vi "Main.vi"(7 "Is Simulated?":bool, 8 "error in":errorcluster, 9 ">>ErrorQ":refnum<queue>, 10 ">>ControllerQ":refnum<queue>, 11 ">>EventHandlers":refnum<user-event>) -> (0 "error out":errorcluster)   [LabVIEW 2020, in "ErrorHandler.lvlib"]
doc: "This is a template for creating new VIs for the owning library"
uses:
  ErrorHandler.lvlib
  Controls/Error QMsg.ctl
  Support/Controls/Project Modules.ctl
  Controller/Controls/Controller QMsg.ctl
  Support/Controls/Project Event Msg.ctl
  Support/Controls/Project Events.ctl
  Controls/Operational Loop Data.ctl
  Support/Support.lvlib
  Controls/Module Event Msg.ctl
  Controller/Controller.lvlib
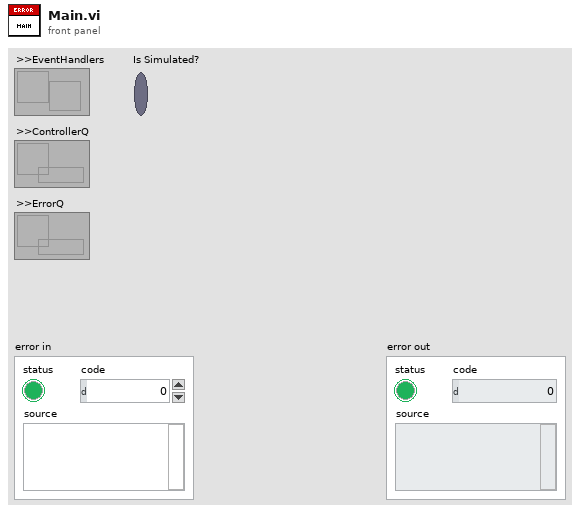
[diagram p1: front panel]
types:
  T1 = typedef "ErrorHandler.lvlib/Operational Loop Data.ctl" = cluster{"Is Simulated?":bool}
  T2 = typedef "ErrorHandler.lvlib/Module Messaging Structures.ctl" = cluster{">>EventHandlers":refnum<user-event>, ">>ErrorQ":refnum<queue>, ">>ControllerQ":refnum<queue>}
  T3 = typedef "ErrorHandler.lvlib/Module Event Msg.ctl" = cluster{"Command":string, "Data":variant}
  T4 = typedef "Support.lvlib/Project Events.ctl" = enum16{"Stop", "Initialize", "Elevator Call"}
  T5 = typedef "Controller.lvlib/Controller QMsg.ctl" = cluster{"Command":string, "Data":variant}
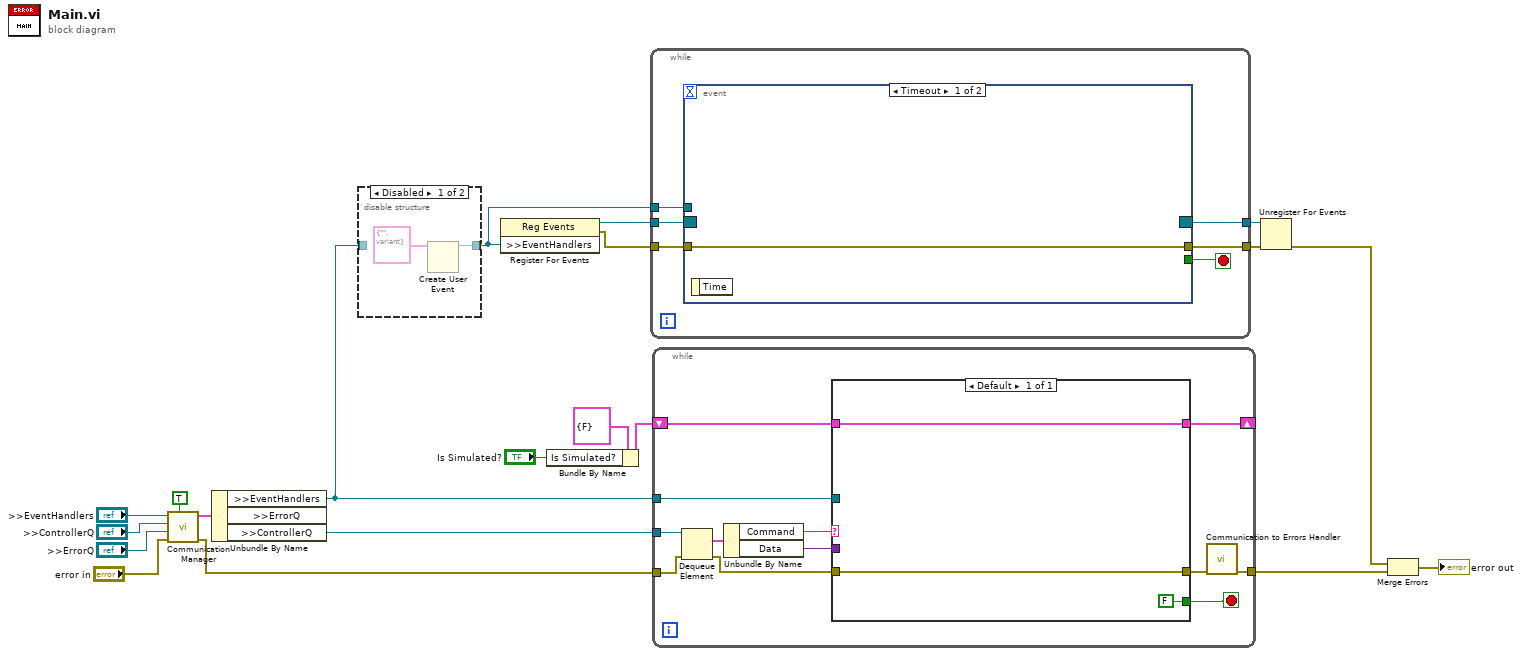
[diagram p0: block diagram]
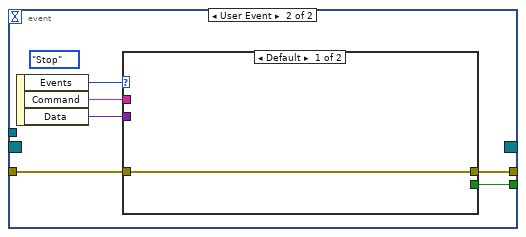
[diagram p3: hidden frame]
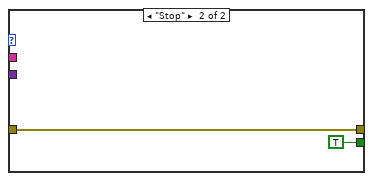
[diagram p4: hidden frame]
diagram:
  n1 = call "Communication Manager.vi"("Load?"=TRUE, "error in"="error in", ">>ErrorQ"=">>ErrorQ", ">>ControllerQ"=">>ControllerQ", ">>EventHandlers"=">>EventHandlers") -> ("error out"=w12:errorcluster, "Messaging Structures"=w15:T2)  [unwired: 5 in]
  n2 = Unbundle By Name(w15) -> (">>EventHandlers"=w2:refnum<user-event>, ">>ControllerQ"=w14:refnum<queue>)  [unwired: 1 out]
  n3 = disable-structure shown="Disabled" {
    disable-tunnel: w2 -> [_ w23]
    disable-tunnel: [w21 w23] -> w1
    frame Disabled {
      n4 = Create User Event(user event datatype=T3 {"Command"="", "Data"=variant} ("QMessage")) -> (user event=w21:refnum<user-event>)  [unwired: 1 in, 1 out]
    }
    frame Enabled {
    }
  }
  n5 = register-events(w1) -> (reference out=w13:refnum<event-registration>, error out=w10:errorcluster)  [unwired: 2 in]
  n6 = Bundle By Name(cluster=T1 {"Is Simulated?"=FALSE} ("Operation Loop Data"), "Is Simulated?"="Is Simulated?") -> (w4:T1)
  n7 = while {
    tunnel: w1 -> [w29]
    tunnel: w13 -> [w28]
    tunnel: [w27] -> w11
    tunnel: w10 -> [w26]
    tunnel: [w25] -> w9
    stop <- w24 stop-if-true
    n8 = event shown="[0] Timeout" {
      selector: w28 -> [_ _]
      dyn-events: [_ _] -> w27
      timeout: _ -> [_ _]
      tunnel: w29 -> [_ _]
      tunnel: w26 -> [w30 w36]
      tunnel: [w30 w35] -> w25
      tunnel: [_ w33] -> w24
      event Timeout {
        n9 = event-data() -> ()  [unwired: 1 in, 1 out]
      }
      event User Event {
        (unwired) Project_Events."Stop" ("Events")
        n10 = event-data() -> ("Events"=w34:T4, "Command"=w32:string, "Data"=w31:variant)  [unwired: 1 in]
        n11 = case shown="Default" w34 {
          tunnel: w36 -> [w37 w39]
          tunnel: [w37 w39] -> w35
          tunnel: [_ TRUE] -> w33
          tunnel: w32 -> [_ _]
          tunnel: w31 -> [_ _]
          frame Default {
          }
          frame "Stop" {
          }
        }
      }
    }
  }
  n12 = while {
    tunnel: w14 -> [w51]
    tunnel: w2 -> [w44]
    tunnel: w12 -> [w50]
    tunnel: [w42] -> w7
    shift-right: [w40] -> _
    shift-left: w4 -> [w41]
    stop <- w46 stop-if-true
    n13 = Dequeue Element(queue=w51, error in (no error)=w50) -> (element=w49:T5, error out=w45:errorcluster)  [unwired: 1 in, 2 out]
    n14 = Unbundle By Name(w49) -> ("Command"=w48:string, "Data"=w47:variant)
    n15 = case shown="Default" w48 {
      tunnel: w47 -> [_]
      tunnel: [FALSE] -> w46
      tunnel: w45 -> [w54]
      tunnel: [w54] -> w43
      tunnel: w44 -> [_]
      tunnel: w41 -> [w53]
      tunnel: [w53] -> w40
      frame Default {
      }
    }
    n16 = call "Communication to Errors Handler.vi"("error in"=w43) -> ("error out"=w42:errorcluster)  [unwired: 10 in]
  }
  n17 = Unregister For Events(event registration refnum=w11, error in=w9) -> (error out=w8:errorcluster)
  n18 = Merge Errors(w8, w7) -> (→"error out":errorcluster)
